vi "读取VISA资源名称.vi"(8 "error in (no error)":errorcluster caption="错误输入（无错误）", 11 "VISA输入":refnum<class "VISA.lvclass">) -> (0 "error out":errorcluster caption="错误输出", 2 "VISA资源名称":refnum<visa-resource-name>, 3 "VISA输出":refnum<class "VISA.lvclass">)   [LabVIEW 2016, in "VISA.lvclass"]
uses:
  VISA.lvclass
  VISA.lvclass/VISA.ctl
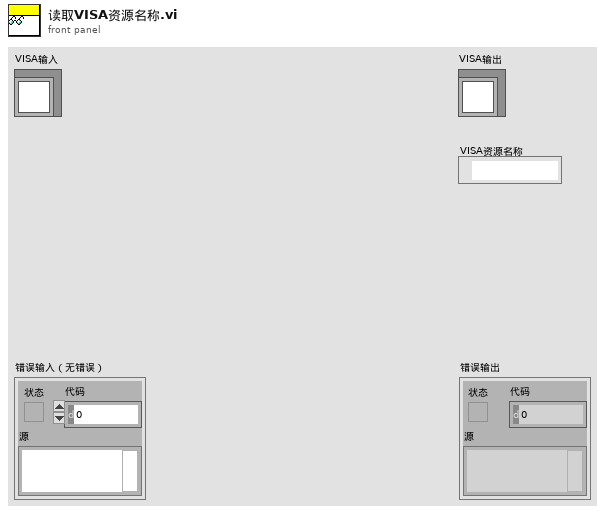
[diagram p1: front panel]
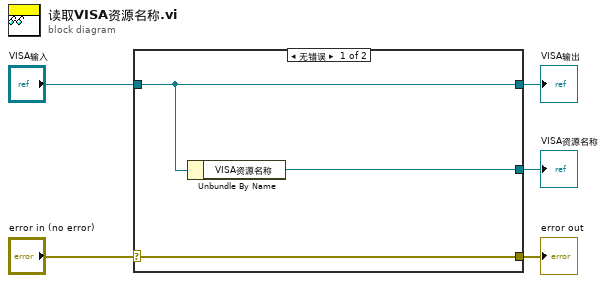
[diagram p0: block diagram]
diagram:
  n1 = case shown="无错误" "error in (no error)" {
    selector: "error in (no error)" -> [w8 w9]
    tunnel: [w8 w9] -> w4
    tunnel: [w7 w10] -> w2
    tunnel: "VISA输入" -> [w7 w10]
    tunnel: [w6 _] -> w1
    frame No Error {
      n2 = Unbundle By Name(w7) -> ("VISA资源名称"=w6:refnum<visa-resource-name>)
    }
    frame Error {
    }
  }
  "error out" <- w4
  "VISA输出" <- w2
  "VISA资源名称" <- w1
